vi "Timer.vi"(8 "error in (no error)":errorcluster, 10 "DigNum Refnum":refnum<vi>, 11 "Notifier in":refnum<notifier>) -> (0 "error out":errorcluster)   [LabVIEW 2014, in "Initialization and IO Node Scripting.lvlib"]
uses:
  Initialization and IO Node Scripting.lvlib
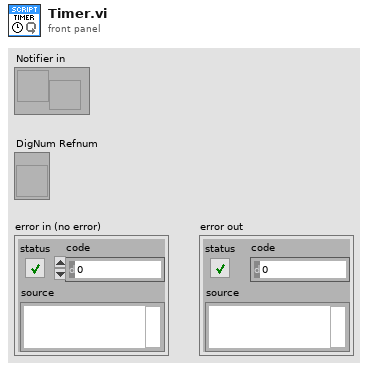
[diagram p1: front panel]
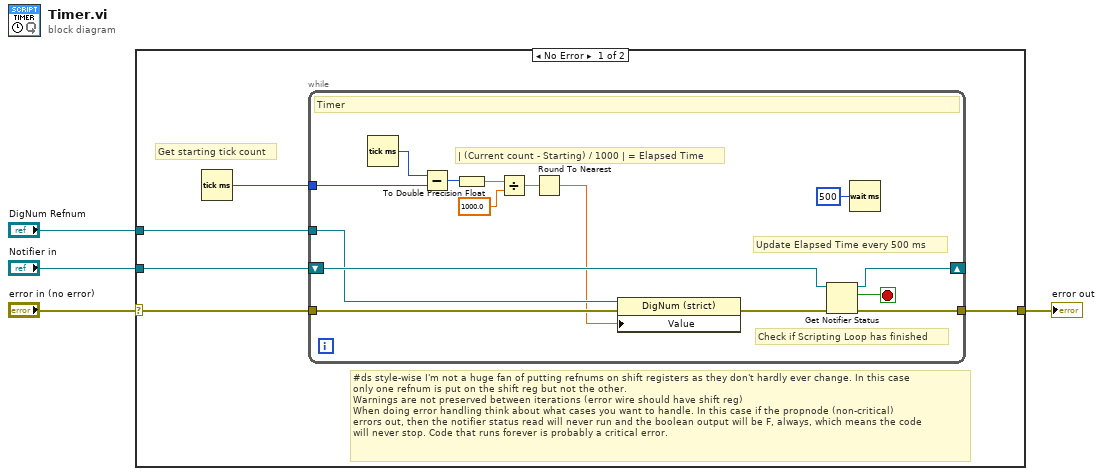
[diagram p0: block diagram]
diagram:
  n1 = case shown="No Error" "error in (no error)" {
    selector: "error in (no error)" -> [w7 w25]
    tunnel: "Notifier in" -> [w9 _]
    tunnel: [w8 w25] -> w3
    tunnel: "DigNum Refnum" -> [w5 _]
    frame No Error {
      # "#ds style-wise I'm not a huge fan of putting refnums on shift registers as they don't hardly ever change. In this case\nonly one refnum is put on the shift reg but not the other.\nWarnings are not preserved between iterations (error wire should have shift reg)\nWhen doing error handling think about what cases you want to handle. In this case if the propnode (non-critical)\nerrors out, then the notifier status read will never run and the boolean output will be F, always, which means the code\nwill never stop. Code that runs forever is probably a critical error."
      # "Get starting tick count"
      n2 = Tick Count (ms)() -> (millisecond timer value=w6:u32)
      n3 = while {
        tunnel: w6 -> [w23]
        tunnel: w7 -> [w13]
        shift-right: [w15] -> _
        shift-left: w9 -> [w17]
        tunnel: [w14] -> w8
        tunnel: w5 -> [w11]
        stop <- w16 stop-if-true
        # "Update Elapsed Time every 500 ms"
        # "| (Current count - Starting) / 1000 | = Elapsed Time"
        # "Check if Scripting Loop has finished"
        # "Timer"
        n4 = Tick Count (ms)() -> (millisecond timer value=w24:u32)
        n5 = Subtract(x=w24, y=w23) -> (x-y=w22:u32)
        n6 = To Double Precision Float(number=w22) -> (double precision float=w21:dbl)
        n7 = Divide(x=w21, y=1000.0) -> (x/y=w19:dbl)
        n8 = Round To Nearest(number=w19) -> (nearest integer value=w10:dbl)
        n9 = property class="DigNum (strict)"(reference=w11, error in=w13, "Value"=w10) -> (error out=w12:errorcluster)  [unwired: 1 out]
        n10 = Get Notifier Status(notifier=w17, error in (no error)=w12) -> (notifier out=w15:refnum<notifier>, current notification=w16:bool, error out=w14:errorcluster)  [unwired: 2 out]
        n11 = Wait (ms)(milliseconds to wait=u32 500) -> ()  [unwired: 1 out]
      }
    }
    frame Error {
    }
  }
  "error out" <- w3
